vi "Program_Active_server.vi"(0 "Client Name":string, 1 "Client Messages":string, 2 "Traverse level State":T1, 3 "Mode":enum16{"Program Active", "Traverse Level State"}(ring), 4 "People to Email":string[](array[string]), 8 "Time till next contact (Sec)":dbl format="%.2f") -> ()   [LabVIEW 2021]
uses:
  ADAM_Global.vi
  ADAM Client/Sub VIs/ADAM Controls/Module_type_ADAM.ctl
  ADAM Client/Sub VIs/ADAM Controls/Function_ADAM.ctl
  ADAM Client/Sub VIs/ADAM Controls/Calib_type_ADAM.ctl
  ADAM Client/Sub VIs/ADAM Controls/Address.ctl
  ADAM Client/Sub VIs/ADAM Controls/Ch_description_ADAM.ctl
  ADAM Client/Sub VIs/ADAM Controls/Channel_State.ctl
  ADAM Client/Sub VIs/ADAM Controls/Traverse_Level_State.ctl
  Anemometry/Anemometry Sub Vis/Globals/Preference_global.vi
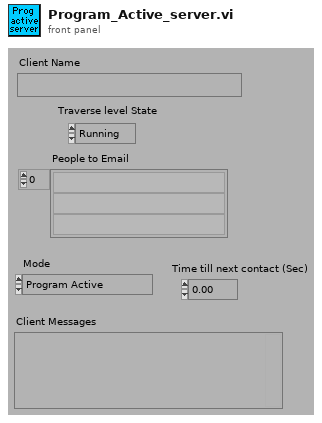
[diagram p1: front panel]
types:
  T1 = typedef "Traverse_Level_State.ctl" = enum16{"Running", "Complete"}
  T2 = typedef "Calib_type_ADAM.ctl" = string
  T3 = typedef "Ch_description_ADAM.ctl" = cluster{"Ch Name":string, "Type":T4, "Function":T5, "Ch State":T6, "Calibration type":T2, "A":dbl, "B":dbl, "C":dbl, "D":dbl, "Comments":string, "Address":T7, "String":string, "Duty":u16}
  T4 = typedef "Module_type_ADAM.ctl" = string
  T5 = typedef "Function_ADAM.ctl" = enum16{"Analogue Input", "Digital Input", "Event counter", "Event rate", "Analogue Output", "Digital Output", "Relay Output"}
  T6 = typedef "Channel_State.ctl" = enum16{"On", "Off", "Always On", "Always Off"}
  T7 = typedef "Address.ctl" = cluster{"Main":i32, "Ch.":i32, "Sub":i32, "Port Name":string}
  T8 = enum16{"Append to Global", "Read Global then Clear"}
  T9 = typedef "Client_State_Cluster.ctl" = cluster{"Client Name":string, "Traverse level State":T1, "People to Email":string[], "Next Contact Time":dbl}
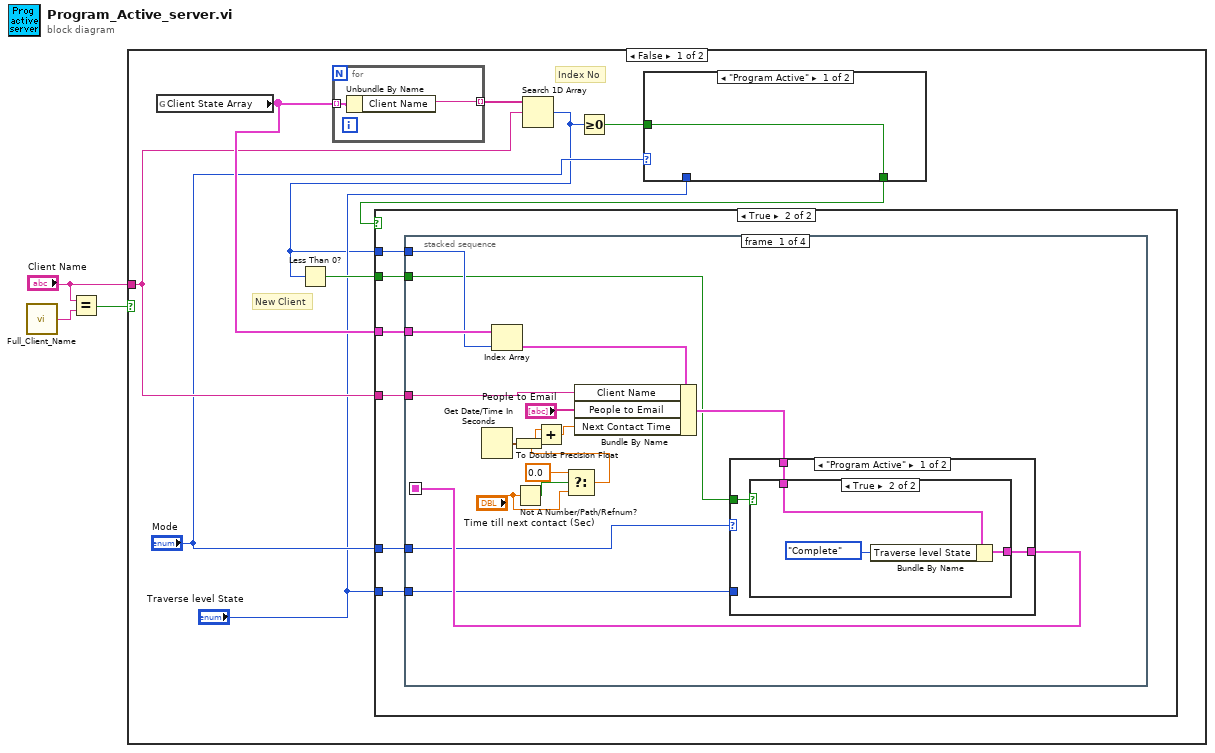
[diagram p0: block diagram]
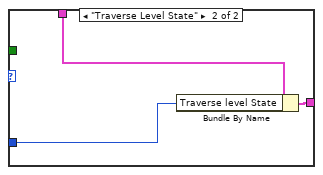
[diagram p4: hidden frame]
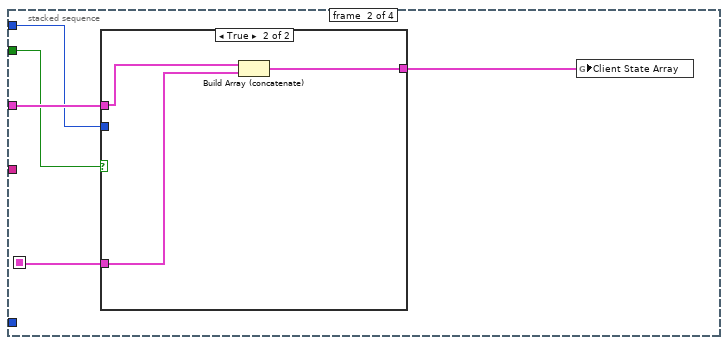
[diagram p5: hidden frame]
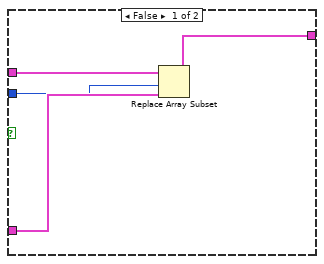
[diagram p6: hidden frame]
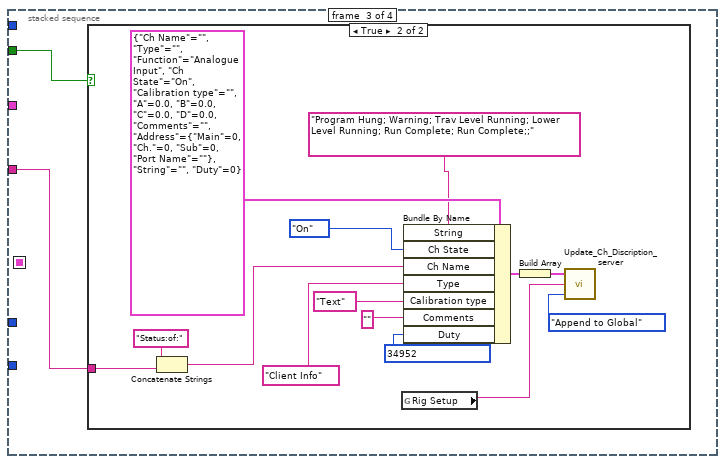
[diagram p7: hidden frame]
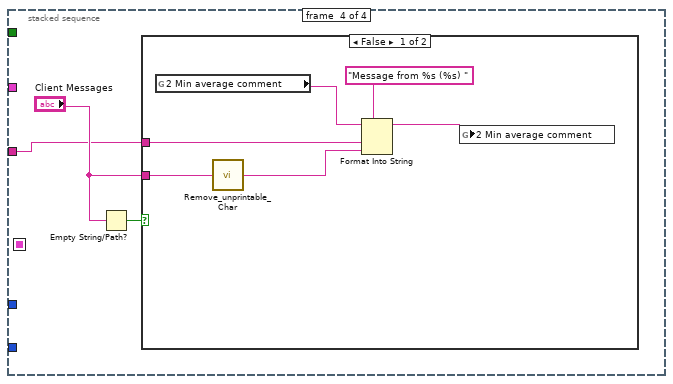
[diagram p9: hidden frame]
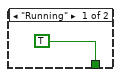
[diagram p12: hidden frame]
diagram:
  n1 = call "Full_Client_Name.vi"() -> ("Client Name"=w2:string)
  n2 = Equal?(x="Client Name", y=w2) -> (x = y?=w1:bool)
  n3 = case shown="False" w1 {
    tunnel: "Client Name" -> [w10 _]
    frame False {
      # "New Client"
      # "Index No"
      n4 = global read "ADAM_Global.vi" "Client State Array"() -> (w12:T9[])
      n5 = for {
        tunnel: w12 -> [w90] mode=indexing
        tunnel: [w89] -> w11 mode=indexing
        n6 = Unbundle By Name(w90) -> ("Client Name"=w89:string)
      }
      n7 = Search 1D Array(1D array=w11, element=w10) -> (index of element=w5:i32)  [unwired: 1 out]
      n8 = Less Than 0?(x=w5) -> (x < 0?=w8:bool)
      n9 = Greater Or Equal To 0?(x=w5) -> (x >= 0?=w4:bool)
      n10 = case shown="\"Program Active\"" "Mode" {
        tunnel: [w83 w86] -> w7
        tunnel: "Traverse level State" -> [_ w85]
        tunnel: w4 -> [w83 w84]
        frame "Program Active" {
        }
        frame "Traverse Level State" {
          n11 = case shown="\"Complete\"" w85 {
            tunnel: [TRUE w88] -> w86
            tunnel: w84 -> [_ w88]
            frame "Running" {
            }
            frame "Complete" {
            }
          }
        }
      }
      n12 = case shown="True" w7 {
        tunnel: "Traverse level State" -> [_ w18]
        tunnel: w12 -> [_ w17]
        tunnel: w10 -> [_ w16]
        tunnel: "Mode" -> [_ w15]
        tunnel: w5 -> [_ w14]
        tunnel: w8 -> [_ w13]
        frame False {
        }
        frame True {
          n13 = stacked-sequence {
            seq-local: [w32 _ _ _] -> [_ w49 _ _]
            tunnel: w17 -> [w35 w50 _ _]
            tunnel: w15 -> [w30 _ _ _]
            tunnel: w18 -> [w29 _ _ _]
            tunnel: w16 -> [w28 _ w59 w74]
            tunnel: w14 -> [w20 w47 _ _]
            tunnel: w13 -> [w19 w46 w58 _]
            frame #0 {
              n14 = Get Date/Time In Seconds() -> (seconds since 1Jan1904=w21:timestamp)
              n15 = Index Array(array=w35, index=w20) -> (element=w34:T9)
              n16 = To Double Precision Float(number=w21) -> (double precision float=w27:dbl)
              n17 = Not A Number/Path/Refnum?(number/path/refnum="Time till next contact (Sec)") -> (NaN/Path/Refnum?=w25:bool)
              n18 = Select(t=0.0, s=w25, f="Time till next contact (Sec)") -> (s? t:f=w22:dbl)
              n19 = Add(x=w27, y=w22) -> (x+y=w26:dbl)
              n20 = Bundle By Name(cluster=w34, "Client Name"=w28, "People to Email"="People to Email", "Next Contact Time"=w26) -> (w33:T9)
              n21 = case shown="\"Program Active\"" w30 {
                tunnel: w33 -> [w37 w45]
                tunnel: [w36 w44] -> w32
                tunnel: w19 -> [w38 _]
                tunnel: w29 -> [_ w43]
                frame "Program Active" {
                  n22 = case shown="True" w38 {
                    tunnel: w37 -> [w39 w42]
                    tunnel: [w39 w41] -> w36
                    frame False {
                    }
                    frame True {
                      n23 = Bundle By Name(cluster=w42, "Traverse level State"=Traverse_Level_State."Complete" ("Bundle Element")) -> (w41:T9)
                    }
                  }
                }
                frame "Traverse Level State" {
                  n24 = Bundle By Name(cluster=w45, "Traverse level State"=w43) -> (w44:T9)
                }
              }
            }
            frame #1 {
              n25 = case shown="True" w46 {
                tunnel: w50 -> [w54 w55]
                tunnel: w49 -> [w52 w57]
                tunnel: [w53 w56] -> w48
                tunnel: w47 -> [w51 _]
                frame False {
                  n26 = Replace Array Subset(array=w54, new element=w52, index=w51) -> (w53:T9[])
                }
                frame True {
                  n27 = Build Array (concatenate)(w55, w57) -> (w56:T9[])
                }
              }
              n28 = global write "ADAM_Global.vi" "Client State Array"(w48) -> ()
            }
            frame #2 {
              n29 = case shown="True" w58 {
                tunnel: w59 -> [_ w64]
                frame False {
                }
                frame True {
                  n30 = Concatenate Strings("Status:of:", w64) -> (w63:string)
                  n31 = global read "Preference_global.vi" "Rig Setup"() -> (w62:string)
                  n32 = Bundle By Name(cluster=T3 {"Ch Name"="", "Type"="", "Function"=enum."Analogue Input", "Ch State"=enum."On", "Calibration type"="", "A"=0.0, "B"=0.0, "C"=0.0, "D"=0.0, "Comments"="", "Address"={"Main"=0, "Ch."=0, "Sub"=0, "Port Name"=""}, "String"="", "Duty"=0} ("Ch Discription"), "String"="Program Hung; Warning; Trav Level Running; Lower Level Running; Run Complete; Run Complete;;", "Ch State"=Channel_State."On", "Ch Name"=w63, "Type"=T4 "Client Info", "Calibration type"=T2 "Text", "Comments"="" ("Substring"), "Duty"=u16 34952 ("Bundle Element")) -> (w72:T3)
                  n33 = Build Array(w72) -> (w71:T3[])
                  n34 = call "Update_Ch_Discription_server.vi"("Mode"=T8."Append to Global", "Client HD name"=w62, "Channels to update In"=w71) -> ()  [unwired: 1 out]
                }
              }
            }
            frame #3 {
              n35 = Empty String/Path?(string/path="Client Messages") -> (empty?=w76:bool)
              n36 = case shown="False" w76 {
                tunnel: "Client Messages" -> [w82 _]
                tunnel: w74 -> [w80 _]
                frame False {
                  n37 = global read "ADAM_Global.vi" "2 Min average comment"() -> (w81:string)
                  n38 = call "Remove_unprintable_Char.vi"("Input String"=w82) -> ("Output String"=w79:string)
                  n39 = Format Into String(format string="Message from %s (%s) ", initial string=w81, w80, w79) -> (resulting string=w77:string)  [unwired: 1 in, 1 out]
                  n40 = global write "ADAM_Global.vi" "2 Min average comment"(w77) -> ()
                }
                frame True {
                }
              }
            }
          }
        }
      }
    }
    frame True {
    }
  }
